vi "Unflatten.vi"(7 "Linked List in":refnum<class "Linked List.lvclass">, 8 "error in (no error)":errorcluster, 9 "Flattened Linked List":string, 10 "Linked List ID":string, 11 "IPersist in":refnum<class "IPersist.lvclass">) -> (0 "error out":errorcluster, 1 "Flattened Linked List out":string, 2 "Linked List ID out":string, 3 "IPersist out":refnum<class "IPersist.lvclass">, 5 "Linked List out":refnum<class "Linked List.lvclass">)   [LabVIEW 2019, in "Linked Lists.lvlib" / "Linked List.lvclass"]
uses:
  <vilib>/gpm_packages/@cs/linked-list/Source/Linked List/Linked List/Linked List.lvclass
  <vilib>/gpm_packages/@cs/persistence/source/IPersist/IPersist.lvclass
  <vilib>/Utility/error.llb/Error Cluster From Error Code.vi
  <vilib>/ErrorRing/Error Ring.xnode
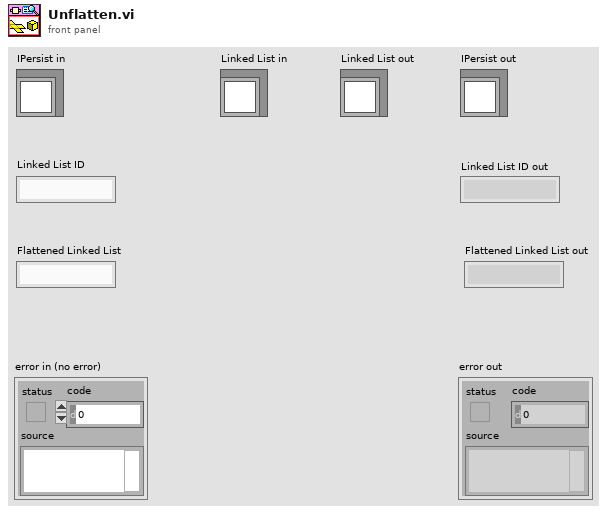
[diagram p1: front panel]
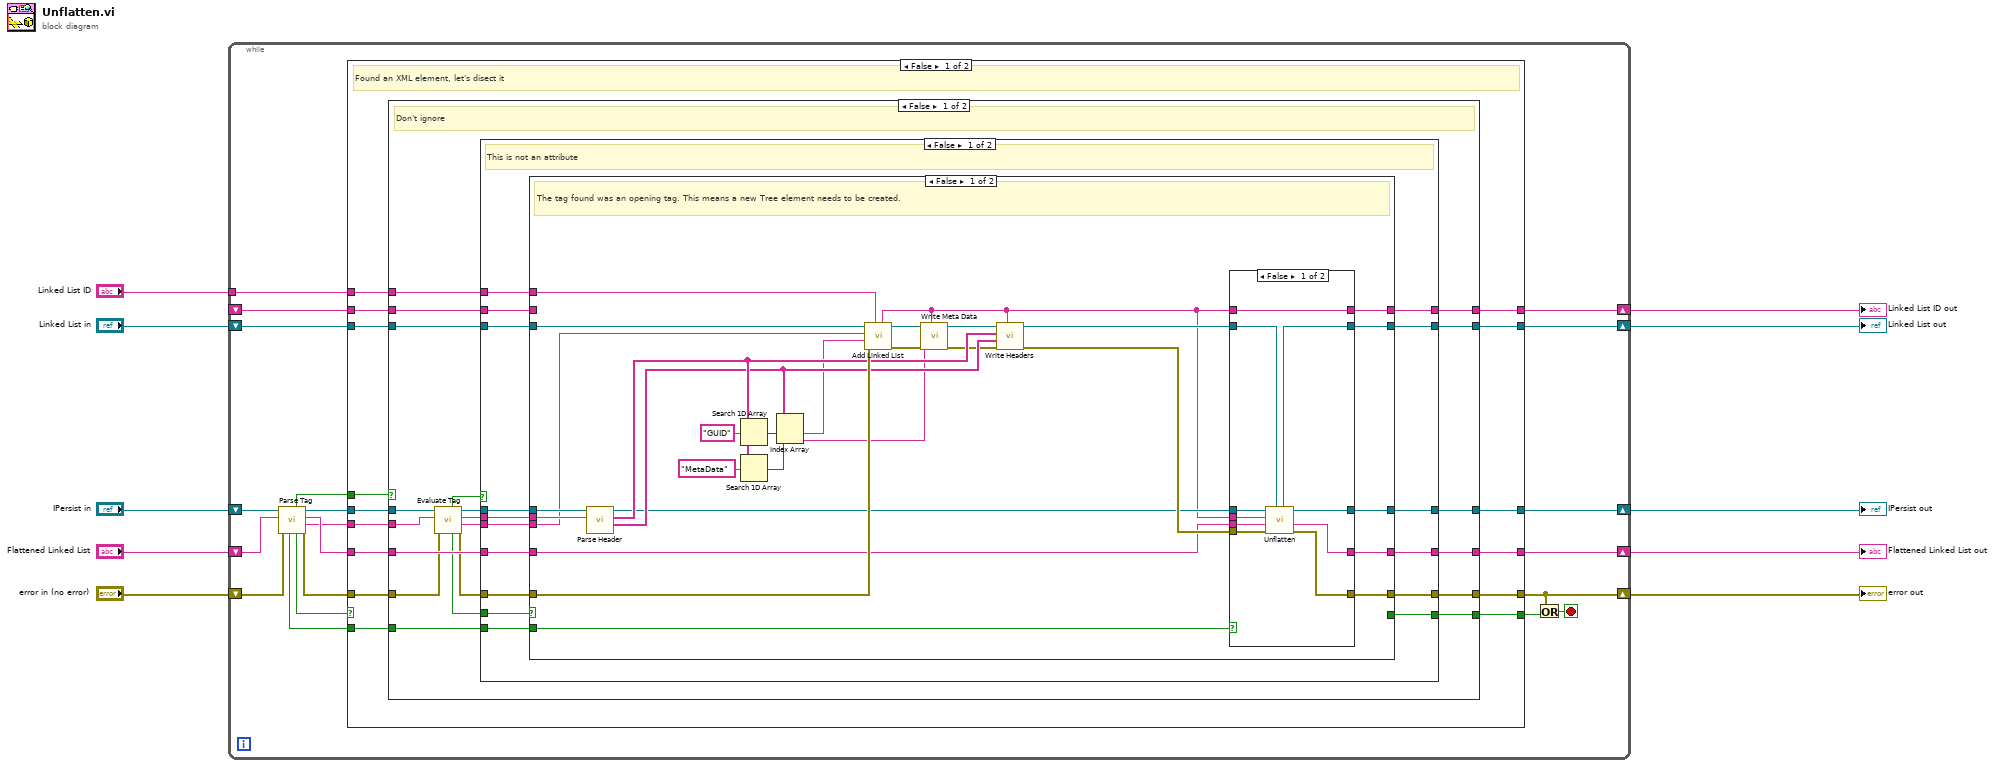
[diagram p0: block diagram]
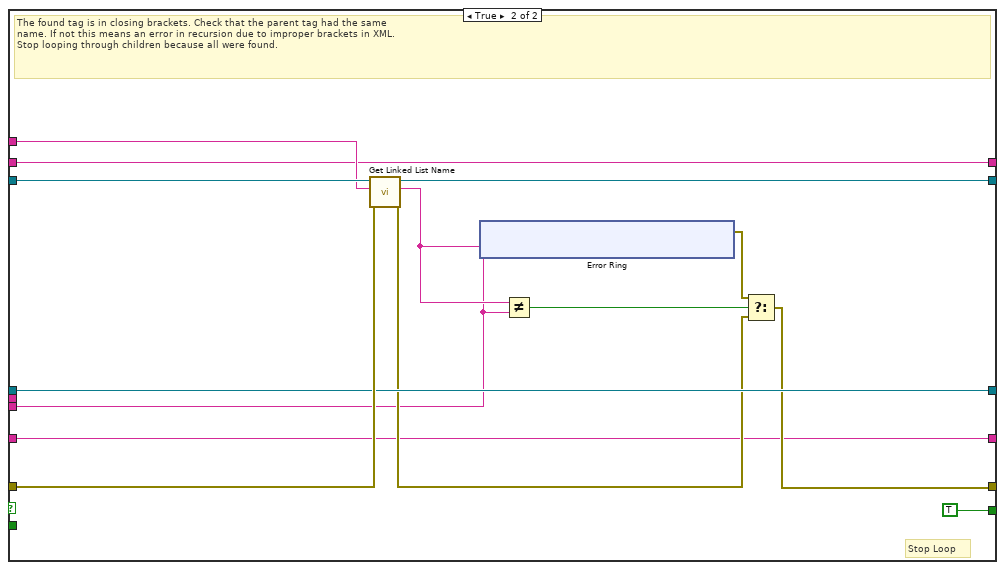
[diagram p3: hidden frame]
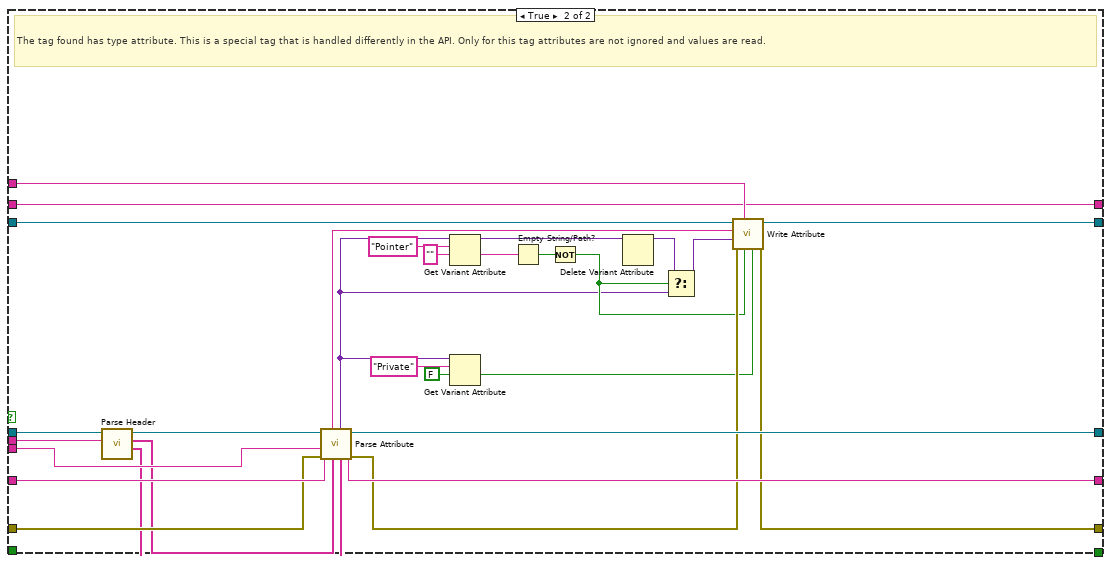
[diagram p4: hidden frame]
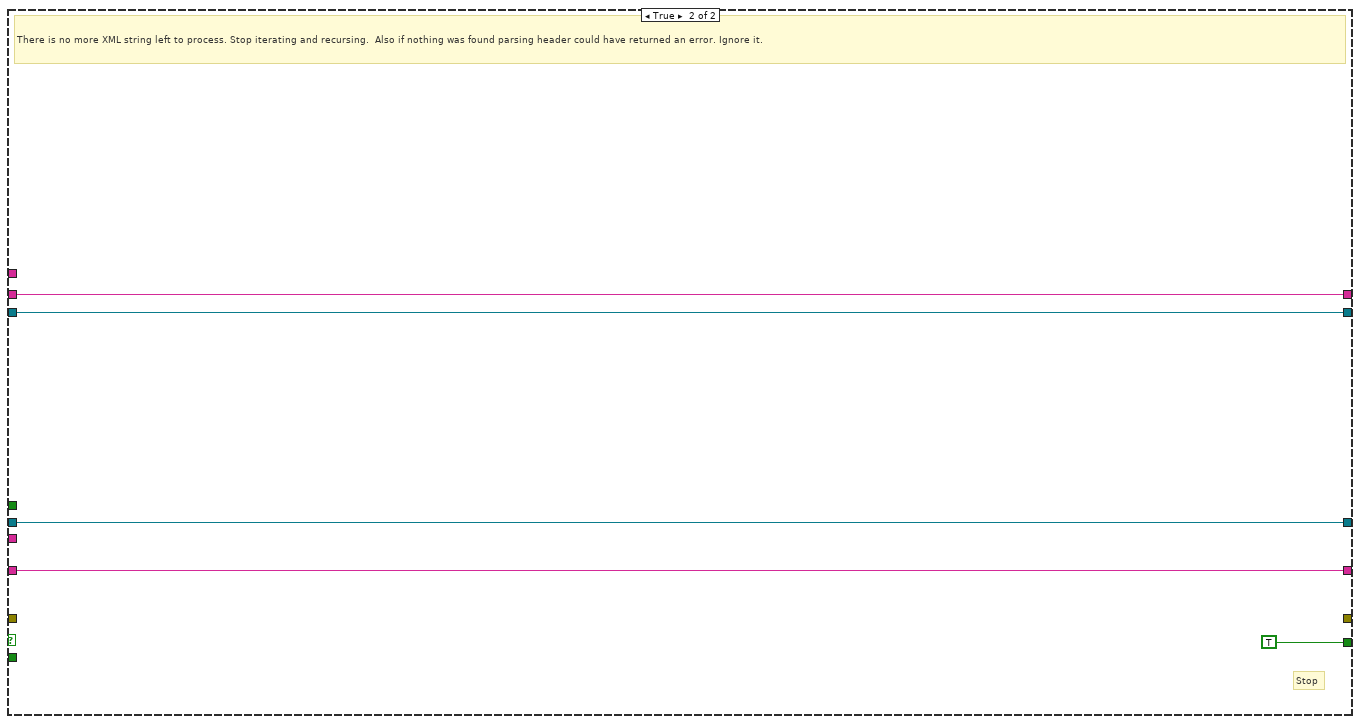
[diagram p6: hidden frame]
diagram:
  n1 = while {
    shift-right: [w29] -> w6
    shift-left: "Linked List in" -> [w30]
    shift-right: [w27] -> w3
    shift-left: "Flattened Linked List" -> [w18]
    shift-right: [w26] -> w5
    shift-left: "error in (no error)" -> [w20]
    shift-right: [w28] -> w1
    shift-left: "IPersist in" -> [w22]
    tunnel: "Linked List ID" -> [w23]
    shift-right: [w14] -> w4
    shift-left: _ -> [w13]
    stop <- w24 stop-if-true
    n2 = call-dynamic "Parse Tag.vi"("error in (no error)"=w20, "Flattened Linked List"=w18, "IPersist in"=w22) -> ("error out"=w19:errorcluster, "Tag"=w12:string, "Flattened Linked List After Tag"=w17:string, "IPersist out"=w21:refnum<class "IPersist.lvclass">, "Nothing Found"=w15:bool, "Ignore"=w16:bool, "Start of Tag"=w11:bool)  [unwired: 2 in]
    n3 = case shown="False" w15 {
      tunnel: w21 -> [w45 w185]
      tunnel: w17 -> [w44 w184]
      tunnel: w19 -> [w43 _]
      tunnel: [w42 _] -> w26
      tunnel: w30 -> [w40 w186]
      tunnel: [w41 w186] -> w29
      tunnel: [w39 w185] -> w28
      tunnel: [w38 w184] -> w27
      tunnel: [w37 TRUE] -> w25
      tunnel: w23 -> [w36 _]
      tunnel: w16 -> [w35 _]
      tunnel: [w34 w182] -> w14
      tunnel: w13 -> [w33 w182]
      tunnel: w12 -> [w32 _]
      tunnel: w11 -> [w31 _]
      frame False {
        # "Found an XML element, let's disect it"
        n4 = case shown="False" w35 {
          tunnel: w45 -> [w55 w179]
          tunnel: w44 -> [w62 w178]
          tunnel: [w60 w181] -> w42
          tunnel: w43 -> [w52 w181]
          tunnel: [w65 w180] -> w41
          tunnel: w40 -> [w64 w180]
          tunnel: [w63 w179] -> w39
          tunnel: [w61 w178] -> w38
          tunnel: [w59 _] -> w37
          tunnel: w36 -> [w58 _]
          tunnel: [w57 w177] -> w34
          tunnel: w33 -> [w56 w177]
          tunnel: w32 -> [w53 _]
          tunnel: w31 -> [w46 _]
          frame False {
            # "Don't ignore"
            n5 = call-dynamic "Evaluate Tag.vi"("error in (no error)"=w52, "Tag"=w53, "IPersist in"=w55) -> ("error out"=w51:errorcluster, "Tag Name"=w48:string, "Header"=w47:string, "IPersist out"=w54:refnum<class "IPersist.lvclass">, "End of Tag"=w49:bool, "Attribute"=w50:bool)  [unwired: 3 in]
            n6 = case shown="False" w50 {
              tunnel: w54 -> [w79 w157]
              tunnel: [w81 w174] -> w65
              tunnel: w64 -> [w80 w175]
              tunnel: [w75 w176] -> w63
              tunnel: w62 -> [w78 w173]
              tunnel: [w72 w172] -> w61
              tunnel: [w74 w170] -> w60
              tunnel: w51 -> [w77 w169]
              tunnel: [w73 _] -> w59
              tunnel: w58 -> [w76 w167]
              tunnel: [w71 w158] -> w57
              tunnel: w56 -> [w70 w158]
              tunnel: w49 -> [w69 _]
              tunnel: w48 -> [w68 w154]
              tunnel: w47 -> [w67 w155]
              tunnel: w46 -> [w66 _]
              frame False {
                # "This is not an attribute"
                n7 = case shown="False" w69 {
                  tunnel: [w106 w138] -> w81
                  tunnel: w80 -> [w110 w139]
                  tunnel: w79 -> [w100 w136]
                  tunnel: w78 -> [w101 w129]
                  tunnel: w77 -> [w109 w137]
                  tunnel: w76 -> [w108 w128]
                  tunnel: [w105 w136] -> w75
                  tunnel: [w103 w131] -> w74
                  tunnel: [_ TRUE] -> w73
                  tunnel: [w102 w129] -> w72
                  tunnel: [w88 w127] -> w71
                  tunnel: w70 -> [_ w127]
                  tunnel: w68 -> [w86 w126]
                  tunnel: w67 -> [w99 _]
                  tunnel: w66 -> [w87 _]
                  frame False {
                    # "The tag found was an opening tag. This means a new Tree element needs to be created."
                    n8 = call-dynamic "Parse Header.vi"("Header"=w99, "IPersist in"=w100) -> ("Value"=w95:string[], "Name"=w96:string[], "IPersist out"=w90:refnum<class "IPersist.lvclass">)  [unwired: 7 in]
                    n9 = Search 1D Array(1D array=w96, element="GUID") -> (index of element=w94:i32)  [unwired: 1 in]
                    n10 = Search 1D Array(1D array=w96, element="MetaData") -> (index of element=w93:i32)  [unwired: 1 in]
                    n11 = Index Array(array=w95, index #1=w94, index #2=w93) -> (element #1=w92:string, element #2=w91:string)
                    n12 = call-dynamic "Add Linked List.vi"("Parent ID"=w108, "error in (no error)"=w109, "Unique ID"=w92, "Name"=w86, "Linked List in"=w110) -> ("error out"=w84:errorcluster, "Linked List out"=w85:refnum<class "Linked List.lvclass">, "Unique ID out"=w89:string)  [unwired: 3 in, 1 out]
                    n13 = call-dynamic "Write Meta Data.vi"("Unique ID"=w89, "error in (no error)"=w84, "Meta Data"=w91, "Linked List in"=w85) -> ("error out"=w82:errorcluster, "Linked List out"=w83:refnum<class "Linked List.lvclass">)  [unwired: 5 in, 1 out]
                    n14 = call-dynamic "Write Headers.vi"("Linked List ID"=w89, "error in (no error)"=w82, "Header Values"=w95, "Header Names"=w96, "Linked List in"=w83) -> ("error out"=w104:errorcluster, "Linked List out"=w107:refnum<class "Linked List.lvclass">)  [unwired: 5 in]
                    n15 = case shown="False" w87 {
                      tunnel: w107 -> [w120 w125]
                      tunnel: [w119 w125] -> w106
                      tunnel: [w118 w123] -> w105
                      tunnel: w104 -> [w117 w121]
                      tunnel: [w116 w121] -> w103
                      tunnel: [w115 w122] -> w102
                      tunnel: w101 -> [w114 w122]
                      tunnel: w89 -> [w113 _]
                      tunnel: w90 -> [w112 w123]
                      tunnel: [w111 w124] -> w88
                      tunnel: w89 -> [w111 w124]
                      frame False {
                        n16 = call-dynamic "Unflatten.vi"("Linked List in"=w120, "error in (no error)"=w117, "Flattened Linked List"=w114, "Linked List ID"=w113, "IPersist in"=w112) -> ("error out"=w116:errorcluster, "Flattened Linked List out"=w115:string, "IPersist out"=w118:refnum<class "IPersist.lvclass">, "Linked List out"=w119:refnum<class "Linked List.lvclass">)  [unwired: 2 in, 1 out]
                      }
                      frame True {
                      }
                    }
                  }
                  frame True {
                    # "Stop Loop"
                    # "The found tag is in closing brackets. Check that the parent tag had the same\nname. If not this means an error in recursion due to improper brackets in XML.\nStop looping through children because all were found."
                    n17 = call-dynamic "Get Linked List Name.vi"("error in (no error)"=w137, "Unique ID"=w128, "Linked List in"=w139) -> ("error out"=w132:errorcluster, "Linked List Name"=w135:string, "Linked List out"=w138:refnum<class "Linked List.lvclass">)  [unwired: 5 in, 1 out]
                    n18 = xnode "Error Ring"("parameter 0"=w135, "parameter 1"=w126) -> ("error out"=w133:errorcluster)
                    n19 = Not Equal?(x=w135, y=w126) -> (x != y?=w134:bool)
                    n20 = Select(t=w133, s=w134, f=w132) -> (s? t:f=w131:errorcluster)
                  }
                }
              }
              frame True {
                # "The tag found has type attribute. This is a special tag that is handled differently in the API. Only for this tag attributes are not ignored and values are read."
                n21 = call-dynamic "Parse Header.vi"("Header"=w155, "IPersist in"=w157) -> ("Value"=w153:string[], "Name"=w152:string[], "IPersist out"=w156:refnum<class "IPersist.lvclass">)  [unwired: 7 in]
                n22 = call-dynamic "Parse Attribute.vi"("Header Values"=w153, "Header Names"=w152, "error in (no error)"=w169, "Tag Name"=w154, "Flattened Linked List"=w173, "IPersist in"=w156) -> ("error out"=w168:errorcluster, "Flattened Linked List out"=w172:string, "IPersist out"=w176:refnum<class "IPersist.lvclass">, "Attribute Value"=w151:variant, "Attribute Name"=w171:string)  [unwired: 1 in]
                n23 = Get Variant Attribute(Variant=w151, name="Pointer", default value (empty Variant)="") -> (duplicate Variant=w164:variant, value=w161:string)  [unwired: 1 in, 2 out]
                n24 = Get Variant Attribute(Variant=w151, name="Private", default value (empty Variant)=FALSE) -> (value=w148:bool)  [unwired: 1 in, 3 out]
                n25 = Empty String/Path?(string/path=w161) -> (empty?=w160:bool)
                n26 = Not(x=w160) -> (.not. x?=w159:bool)
                n27 = Delete Variant Attribute(7:w164) -> (3:w163:variant)  [unwired: 2 in, 2 out]
                n28 = Select(t=w163, s=w159, f=w151) -> (s? t:f=w162:variant)
                n29 = call-dynamic "Write Attribute.vi"("Private?"=w148, "Pointer?"=w159, "Linked List ID"=w167, "error in (no error)"=w168, "Attribute"=w162, "Attribute Name"=w171, "Linked List in"=w175) -> ("error out"=w170:errorcluster, "Linked List out"=w174:refnum<class "Linked List.lvclass">)  [unwired: 1 in, 2 out]
              }
            }
          }
          frame True {
            # "Ignore this element due to syntax of header"
          }
        }
      }
      frame True {
        # "Stop"
        # "There is no more XML string left to process. Stop iterating and recursing.  Also if nothing was found parsing header could have returned an error. Ignore it."
      }
    }
    n30 = Or(x=w26, y=w25) -> (x .or. y?=w24:bool)
  }
  "error out" <- w5
  "Linked List out" <- w6
  "IPersist out" <- w1
  "Flattened Linked List out" <- w3
  "Linked List ID out" <- w4
